vi "PathPlanner_GeomUtil_CoerceHeadingRadians.vi"(11 "in Radians":dbl) -> (3 "out Radians":dbl)   [LabVIEW 2019, in "PathPlanner.lvlib"]
uses:
  PathPlanner.lvlib
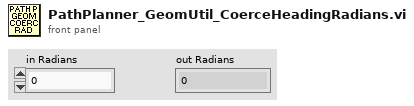
[diagram p1: front panel]
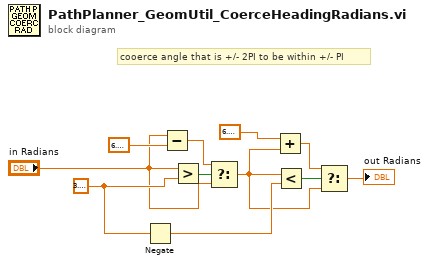
[diagram p0: block diagram]
diagram:
  w8 = 3.141592653589793
  # "cooerce angle that is +/- 2PI to be within +/- PI"
  n1 = Negate(x=w8) -> (-x=w7:dbl)
  n2 = Subtract(x="in Radians", y=6.283185307179586) -> (x-y=w10:dbl)
  n3 = Greater?(x="in Radians", y=w8) -> (0:w11:bool)
  n4 = Select(t=w10, s=w11, f="in Radians") -> (s? t:f=w5:dbl)
  n5 = Add(x=6.283185307179586, y=w5) -> (x+y=w4:dbl)
  n6 = Less?(x=w5, y=w7) -> (x < y?=w6:bool)
  n7 = Select(t=w4, s=w6, f=w5) -> (s? t:f=→"out Radians":dbl)
